vi "Main.vi"() -> ()   [LabVIEW 2019]
uses:
  Type Definitions/Machine States/Signal Playback State.ctl
  Type Definitions/Machine States/Oscillator State.ctl
  Type Definitions/UI.ctl
  Type Definitions/UIOscillatorParam.ctl
  Type Definitions/Sub Oscillalator Type.ctl
  Type Definitions/UIADSRParam.ctl
  Type Definitions/UILowpassParam.ctl
  Type Definitions/UITremolo.ctl
  Type Definitions/DataInOut.ctl
  <vilib>/sound2/lvsound2.llb/Sampling Mode.ctl
  <vilib>/sound2/lvsound2.llb/Sound Data Format.ctl
  <vilib>/sound2/lvsound2.llb/Sound Output Set Volume (Single).vi
  <vilib>/sound2/lvsound2.llb/Sound Output Write (DBL Single).vi
panel:
  in  "Cluster":T1={"oscillator"={"signal type"=0, "pulse width"=0.0, "Sub oscillator"=enum."Off", "Frequency"=0.0, "Amplitude"=0.0}, "ADSR"={"A"=0, "D"=0, "S"=0, "R"=0, "volume"=0.0}, "Lowpass filter"={"Lowpass on/off"=FALSE, "Cutoff frequency"=20.0}, "Tremolo"={"Rate"=0.0, "LFO frequency"=20.0, " on/off "=FALSE}} {"Tremolo"."LFO frequency" min=0.0 max=25.0 scale=0.0..25.0; "Tremolo"."Rate" min=0.0 max=1.0 scale=0.0..1.0; "Lowpass filter"."Cutoff frequency" min=20.0 max=20000.0 scale=20.0..20000.0; "ADSR"."volume" min=0.0 max=100.0 scale=0.0..100.0; "ADSR"."R" scale=0.0..100.0; "ADSR"."S" scale=0.0..100.0; "ADSR"."D" scale=0.0..100.0; "ADSR"."A" scale=0.0..100.0; "oscillator"."Amplitude" scale=0.0..10.0; "oscillator"."Frequency" scale=0.0..10.0; "oscillator"."pulse width" min=0.0 max=100.0 scale=0.0..100.0; "oscillator"."signal type" items=["Sine Wave", "Triangle Wave", "Square Wave", "Sawtooth Wave"]}
  out "Enum":T7
  in  "Sound button":bool
  out "element":waveform(dbl)(graph)
  out "Play State":T8
  out "# elements in queue":i32
  in  "Play Button":bool
  in  "Stop Button":bool
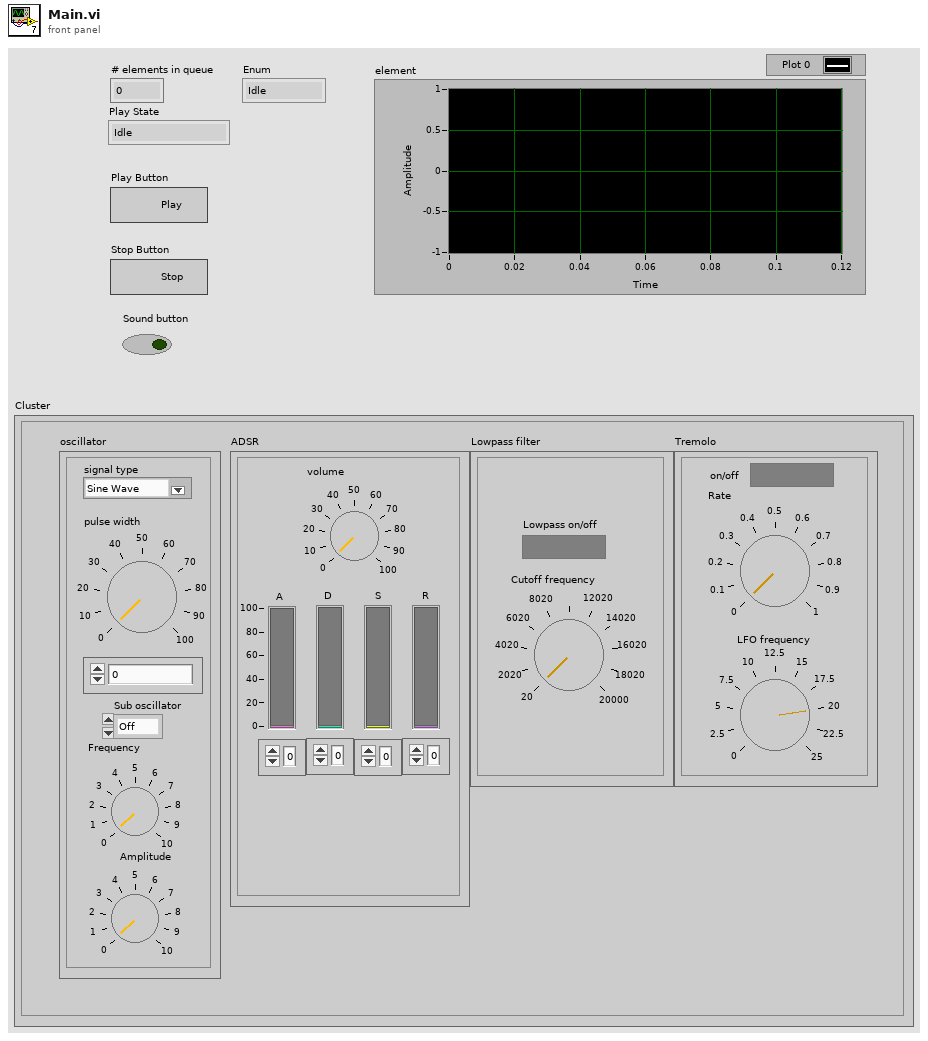
[diagram p1: front panel]
types:
  T1 = typedef "UI.ctl" = cluster{"oscillator":T2, "ADSR":T4, "Lowpass filter":T5, "Tremolo":T6}
  T2 = typedef "UIOscillatorParam.ctl" = cluster{"signal type":u16, "pulse width":dbl, "Sub oscillator":T3, "Frequency":dbl, "Amplitude":dbl}
  T3 = typedef "Sub Oscillalator Type.ctl" = enum16{"Off", "One Octave", "Two Octaves"}
  T4 = typedef "UIADSRParam.ctl" = cluster{"A":i32, "D":i32, "S":i32, "R":i32, "volume":dbl}
  T5 = typedef "UILowpassParam.ctl" = cluster{"Lowpass on/off":bool, "Cutoff frequency":dbl}
  T6 = typedef "UITremolo.ctl" = cluster{"Rate":dbl, "LFO frequency":dbl, " on/off ":bool}
  T7 = typedef "Oscillator State.ctl" = enum16{"Idle", "Attack", "Decay", "Sustain", "Release"}
  T8 = typedef "Signal Playback State.ctl" = enum16{"Idle", "Initialization", "Playing", "End"}
  T9 = typedef "DataInOut.ctl" = enum16{"write", "read"}
  T10 = typedef "Sound Data Format.ctl" = cluster{"sample rate (S/s)":dbl, "number of channels":i32, "bits per sample":i32}
  T11 = typedef "Sampling Mode.ctl" = i32
  T12 = typedef "Sound Output Task ID.ctl" = u32
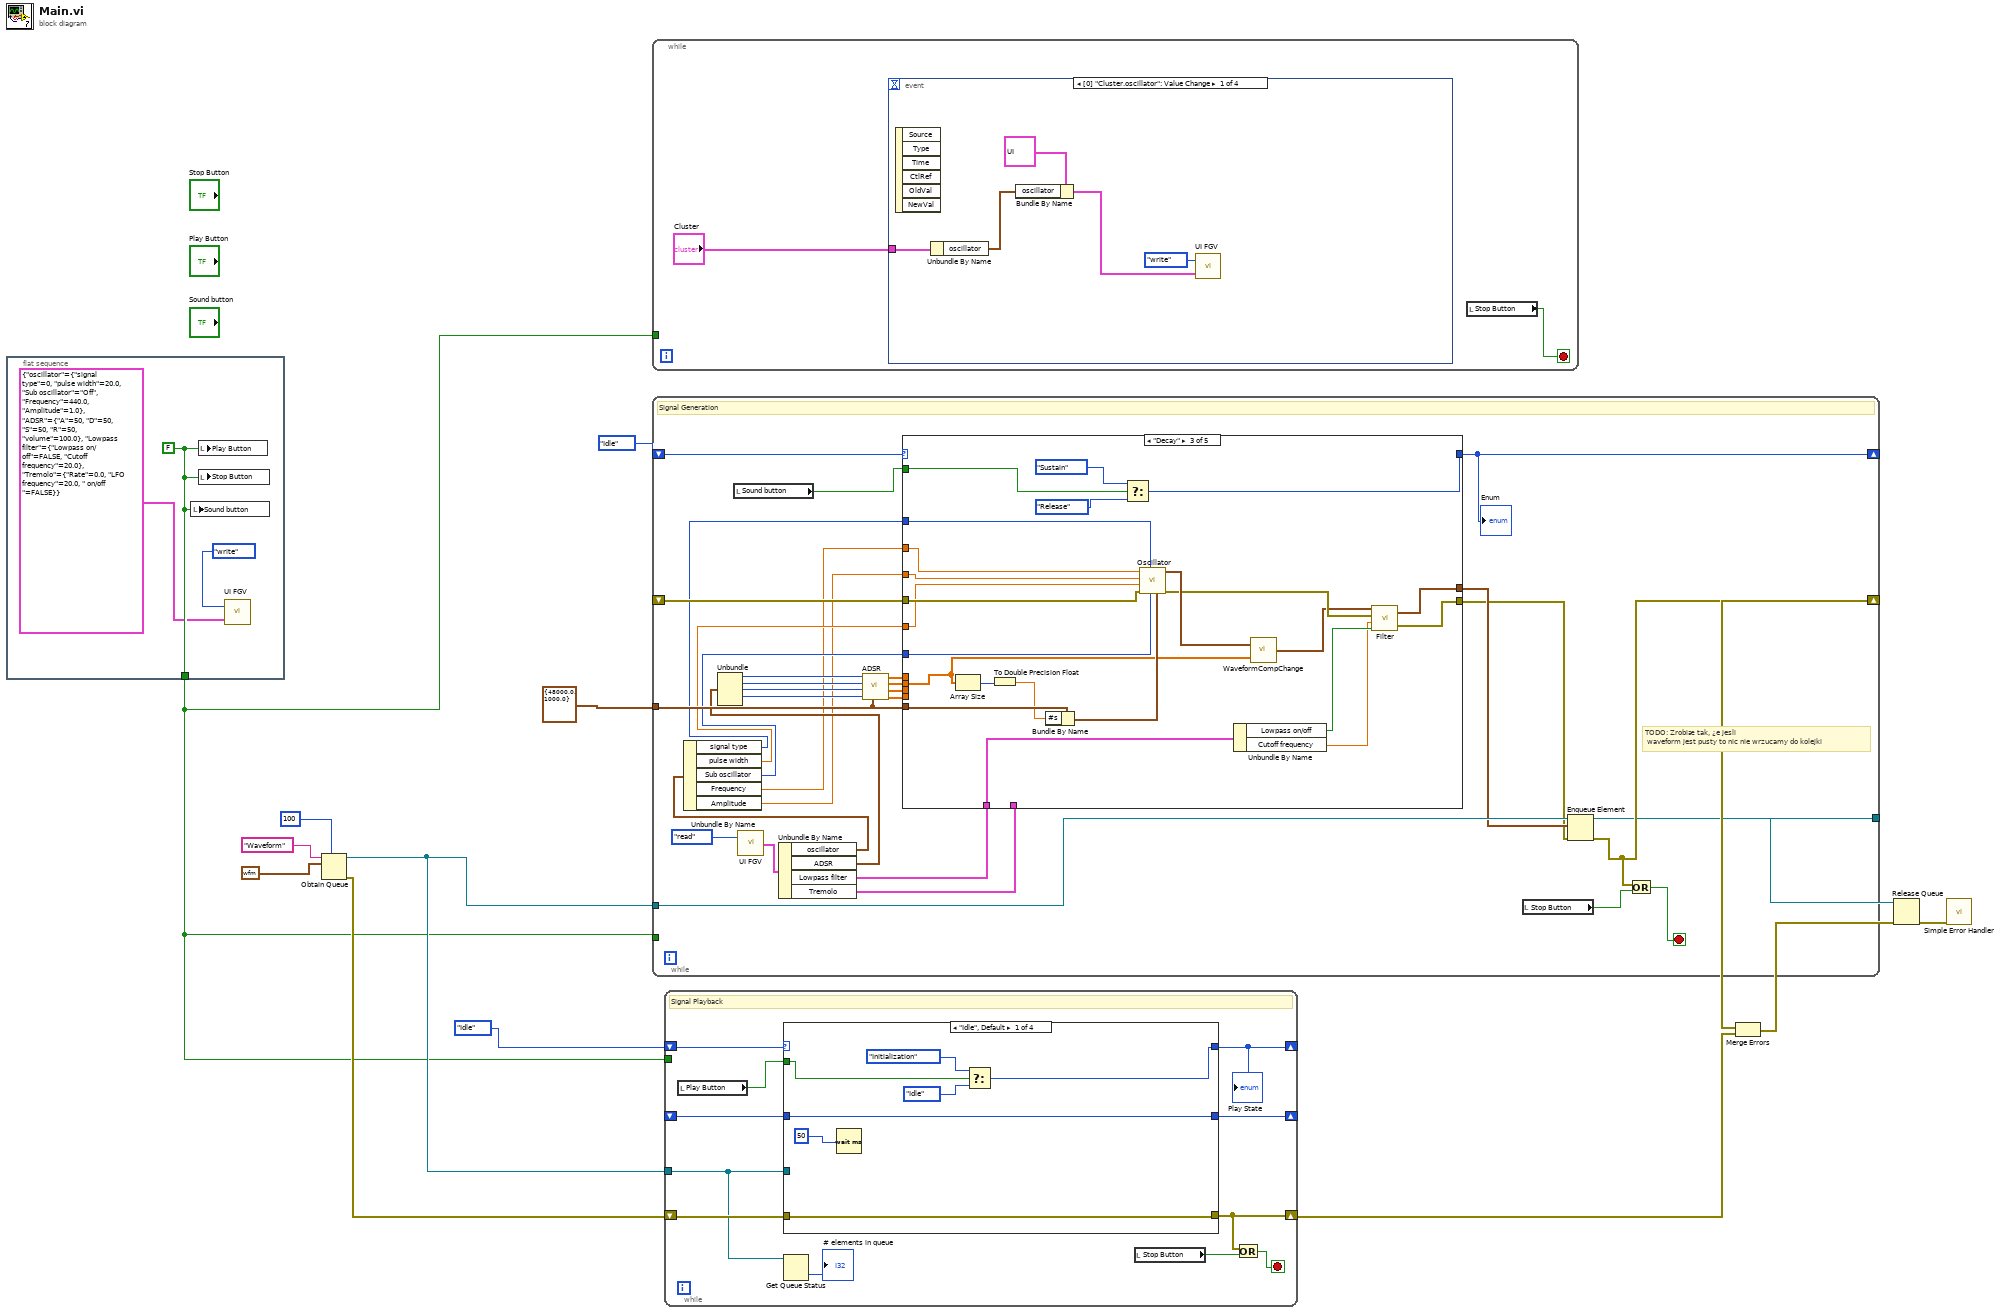
[diagram p0: block diagram]
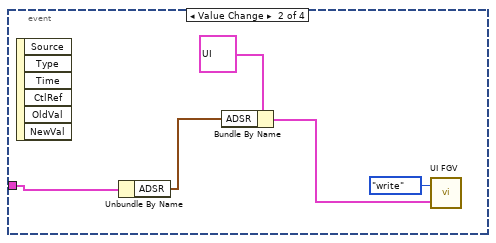
[diagram p2: hidden frame]
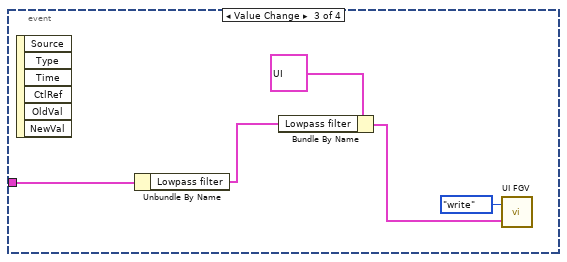
[diagram p3: hidden frame]
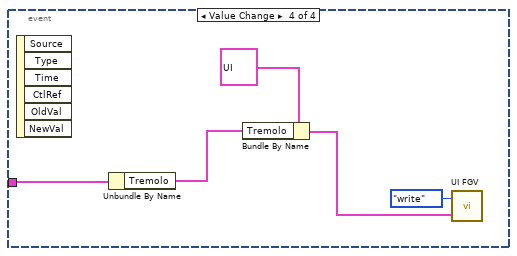
[diagram p4: hidden frame]
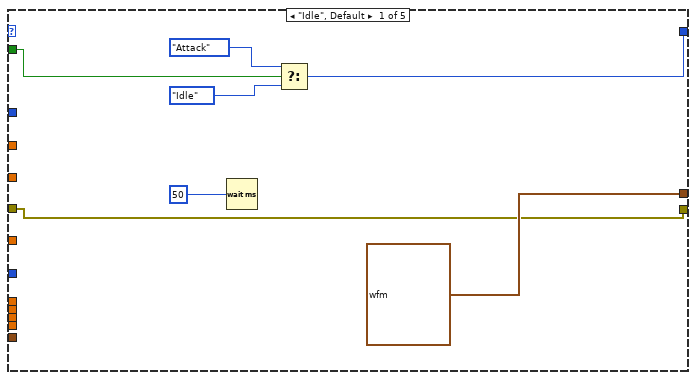
[diagram p5: hidden frame]
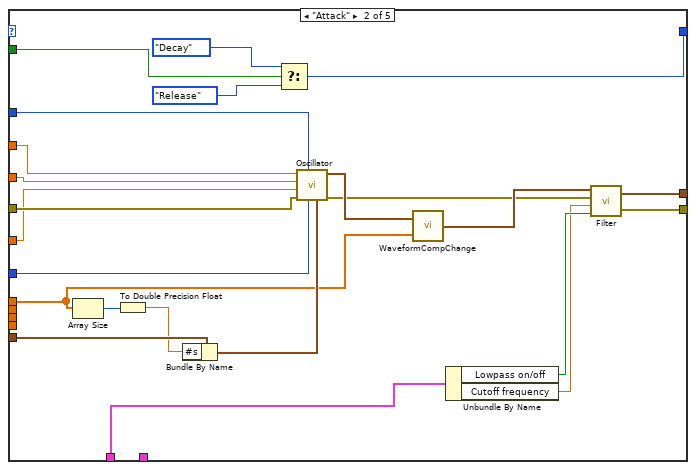
[diagram p6: hidden frame]
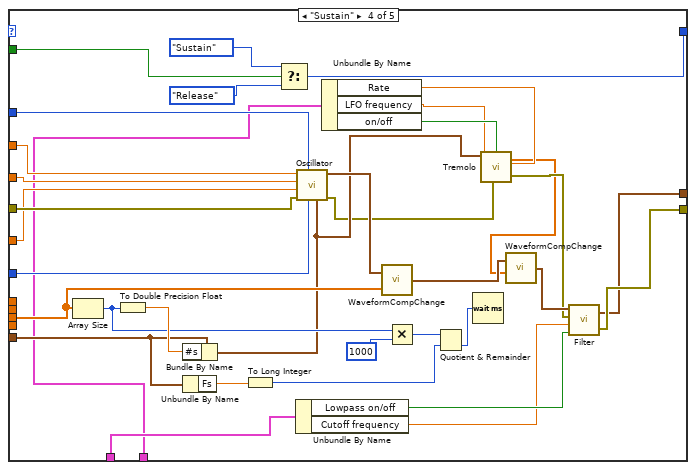
[diagram p7: hidden frame]
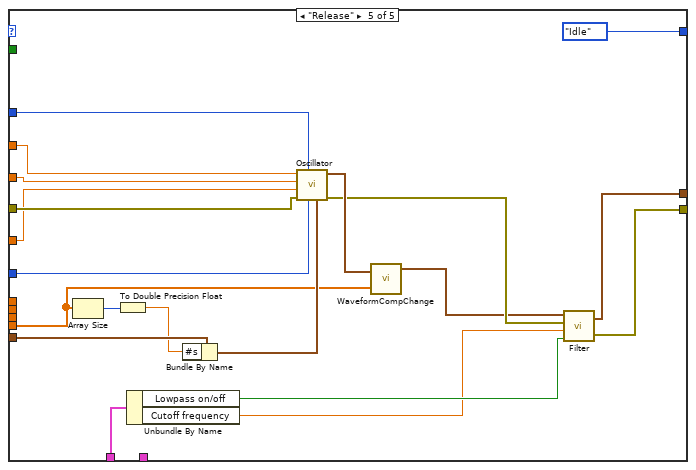
[diagram p8: hidden frame]
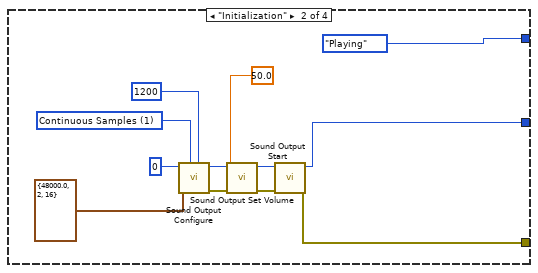
[diagram p9: hidden frame]
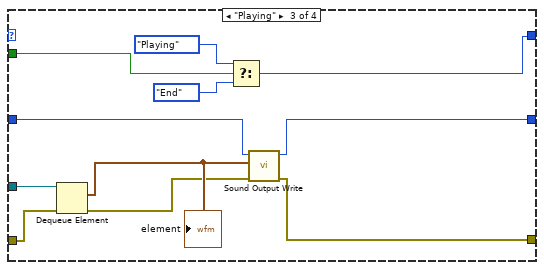
[diagram p10: hidden frame]
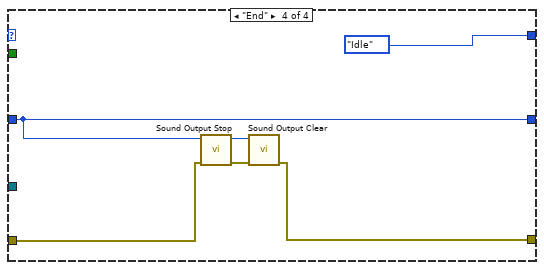
[diagram p11: hidden frame]
diagram:
  n1 = flat-sequence {
    tunnel: [w17] -> w1
    frame #0 {
      w17 = FALSE ("Play Button")
      n2 = local write "Sound button"(w17) -> ()
      n3 = local write "Play Button"(w17) -> ()
      n4 = local write "Stop Button"(w17) -> ()
      n5 = call "UI FGV.vi"("Data in"=T1 {"oscillator"={"signal type"=0, "pulse width"=20.0, "Sub oscillator"=enum."Off", "Frequency"=440.0, "Amplitude"=1.0}, "ADSR"={"A"=50, "D"=50, "S"=50, "R"=50, "volume"=100.0}, "Lowpass filter"={"Lowpass on/off"=FALSE, "Cutoff frequency"=20.0}, "Tremolo"={"Rate"=0.0, "LFO frequency"=20.0, " on/off "=FALSE}}, "Enum"=DataInOut."write") -> ()  [unwired: 1 out]
    }
  }
  n6 = Obtain Queue(max queue size (-1, unlimited)=100, name (unnamed)="Waveform", element data type=waveform(dbl) {"t0"=timestamp(0 s since 1904-01-01), "dt"=1.0, "Y"=[]} ("Waveform out")) -> (queue out=w4:refnum<queue>, error out=w12:errorcluster)  [unwired: 2 in, 1 out]
  n7 = while "User Interface" {
    tunnel: w1 -> [_]
    stop <- w18 stop-if-true
    n8 = event shown="[0] \"Cluster.oscillator\": Value Change" {
      selector: _ -> [_ _ _ _]
      dyn-events: _ -> [_ _ _ _]
      timeout: _ -> [_ _ _ _]
      tunnel: "Cluster" -> [w21 w26 w31 w35]
      event Value Change {
        n9 = event-data() -> ()  [unwired: 1 in, 6 out]
        n10 = Unbundle By Name(w21) -> ("oscillator"=w20:T2)
        n11 = Bundle By Name(cluster=T1 {"oscillator"={"signal type"=0, "pulse width"=0.0, "Sub oscillator"=enum."Off", "Frequency"=0.0, "Amplitude"=0.0}, "ADSR"={"A"=0, "D"=0, "S"=0, "R"=0, "volume"=0.0}, "Lowpass filter"={"Lowpass on/off"=FALSE, "Cutoff frequency"=20.0}, "Tremolo"={"Rate"=0.0, "LFO frequency"=20.0, " on/off "=FALSE}} ("Data in"), "oscillator"=w20) -> (w22:T1)
        n12 = call "UI FGV.vi"("Data in"=w22, "Enum"=DataInOut."write") -> ()  [unwired: 1 out]
      }
      event Value Change {
        n13 = event-data() -> ()  [unwired: 1 in, 6 out]
        n14 = Unbundle By Name(w26) -> ("ADSR"=w25:T4)
        n15 = Bundle By Name(cluster=T1 {"oscillator"={"signal type"=0, "pulse width"=0.0, "Sub oscillator"=enum."Off", "Frequency"=0.0, "Amplitude"=0.0}, "ADSR"={"A"=0, "D"=0, "S"=0, "R"=0, "volume"=0.0}, "Lowpass filter"={"Lowpass on/off"=FALSE, "Cutoff frequency"=20.0}, "Tremolo"={"Rate"=0.0, "LFO frequency"=20.0, " on/off "=FALSE}} ("Data in"), "ADSR"=w25) -> (w27:T1)
        n16 = call "UI FGV.vi"("Data in"=w27, "Enum"=DataInOut."write") -> ()  [unwired: 1 out]
      }
      event Value Change {
        n17 = event-data() -> ()  [unwired: 1 in, 6 out]
        n18 = Unbundle By Name(w31) -> ("Lowpass filter"=w30:T5)
        n19 = Bundle By Name(cluster=T1 {"oscillator"={"signal type"=0, "pulse width"=0.0, "Sub oscillator"=enum."Off", "Frequency"=0.0, "Amplitude"=0.0}, "ADSR"={"A"=0, "D"=0, "S"=0, "R"=0, "volume"=0.0}, "Lowpass filter"={"Lowpass on/off"=FALSE, "Cutoff frequency"=20.0}, "Tremolo"={"Rate"=0.0, "LFO frequency"=20.0, " on/off "=FALSE}} ("Data in"), "Lowpass filter"=w30) -> (w32:T1)
        n20 = call "UI FGV.vi"("Data in"=w32, "Enum"=DataInOut."write") -> ()  [unwired: 1 out]
      }
      event Value Change {
        n21 = event-data() -> ()  [unwired: 1 in, 6 out]
        n22 = Unbundle By Name(w35) -> ("Tremolo"=w36:T6)
        n23 = Bundle By Name(cluster=T1 {"oscillator"={"signal type"=0, "pulse width"=0.0, "Sub oscillator"=enum."Off", "Frequency"=0.0, "Amplitude"=0.0}, "ADSR"={"A"=0, "D"=0, "S"=0, "R"=0, "volume"=0.0}, "Lowpass filter"={"Lowpass on/off"=FALSE, "Cutoff frequency"=20.0}, "Tremolo"={"Rate"=0.0, "LFO frequency"=20.0, " on/off "=FALSE}} ("Data in"), "Tremolo"=w36) -> (w37:T1)
        n24 = call "UI FGV.vi"("Data in"=w37, "Enum"=DataInOut."write") -> ()  [unwired: 1 out]
      }
    }
    n25 = local read "Stop Button"() -> (w18:bool)
  }
  n26 = while {
    shift-right: [w68] -> _
    shift-left: Oscillator_State."Idle" -> [w70]
    tunnel: cluster{"Fs":dbl, "#s":dbl} {"Fs"=48000.0, "#s"=1000.0} ("Sampling info") -> [w62]
    shift-right: [w64] -> w2
    shift-left: _ -> [w69]
    tunnel: w1 -> [_]
    tunnel: w4 -> [w53]
    tunnel: [w63] -> w3
    stop <- w65 stop-if-true
    # "TODO: Zrobiæ tak, ¿e jesli\n waveform jest pusty to nic nie wrzucamy do kolejki"
    # "Signal Generation"
    n27 = local read "Sound button"() -> (w67:bool)
    n28 = call "UI FGV.vi"("Enum"=DataInOut."read") -> ("Data out"=w49:T1)  [unwired: 1 in]
    n29 = Unbundle By Name(w49) -> ("oscillator"=w48:T2, "ADSR"=w44:T4, "Lowpass filter"=w43:T5, "Tremolo"=w42:T6)
    n30 = Unbundle By Name(w48) -> ("signal type"=w47:u16, "pulse width"=w46:dbl, "Sub oscillator"=w45:T3, "Frequency"=w41:dbl, "Amplitude"=w40:dbl)
    n31 = Unbundle(w44) -> ("A"=w61:i32, "D"=w60:i32, "S"=w59:i32, "R"=w58:i32)  [unwired: 1 out]
    n32 = call "ADSR.vi"("Sampling info"=w62, "R"=w58, "S"=w59, "D"=w60, "A"=w61) -> ("R"=w54:dbl[], "S"=w55:dbl[], "D"=w56:dbl[], "A"=w57:dbl[])  [unwired: 3 in]
    n33 = case shown="\"Decay\"" w70 {
      tunnel: [w75 w99 w121 w156 Oscillator_State."Idle"] -> w68
      tunnel: w67 -> [w73 w98 w120 w155 _]
      tunnel: w47 -> [_ w92 w114 w149 w173]
      tunnel: w41 -> [_ w93 w115 w150 w174]
      tunnel: w40 -> [_ w94 w116 w151 w175]
      tunnel: w69 -> [w71 w97 w119 w154 w178]
      tunnel: w46 -> [_ w96 w118 w153 w177]
      tunnel: w45 -> [_ w95 w117 w152 w176]
      tunnel: w62 -> [_ w91 w113 w145 w172]
      tunnel: [w71 w79 w102 w132 w159] -> w51
      tunnel: [waveform(dbl) {"t0"=timestamp(0 s since 1904-01-01), "dt"=1.0, "Y"=[]} ("signal out") w78 w101 w131 w160] -> w52
      tunnel: w57 -> [_ w86 _ _ _]
      tunnel: w56 -> [_ _ w108 _ _]
      tunnel: w55 -> [_ _ _ w139 _]
      tunnel: w54 -> [_ _ _ _ w166]
      tunnel: w43 -> [_ w84 w107 w137 w165]
      tunnel: w42 -> [_ _ _ w136 _]
      frame "Idle", Default {
        n34 = Wait (ms)(milliseconds to wait=u32 50) -> ()  [unwired: 1 out]
        n35 = Select(t=Oscillator_State."Attack", s=w73, f=Oscillator_State."Idle") -> (s? t:f=w75:T7)
      }
      frame "Attack" {
        n36 = Array Size(array=w86) -> (size(s)=w90:i32)
        n37 = To Double Precision Float(number=w90) -> (double precision float=w89:dbl)
        n38 = Bundle By Name(cluster=w91, "#s"=w89) -> (w88:cluster{"Fs":dbl, "#s":dbl})
        n39 = Select(t=Oscillator_State."Decay", s=w98, f=Oscillator_State."Release") -> (s? t:f=w99:T7)
        n40 = call "Oscillator.vi"("Sampling info"=w88, "Sub Oscillator Type"=w95, "Waveform type"=w92, "Error in"=w97, "Pulse Width"=w96, "Amplitude"=w94, "Frequency"=w93) -> ("Error out"=w80:errorcluster, "Waveform out"=w85:waveform(dbl))  [unwired: 3 in]
        n41 = call "WaveformCompChange.vi"("component"=w86, "input waveform"=w85) -> ("output waveform"=w81:waveform(dbl))
        n42 = Unbundle By Name(w84) -> ("Lowpass on/off"=w83:bool, "Cutoff frequency"=w82:dbl)
        n43 = call "Filter.vi"("on/off"=w83, "Cutoff freq (Hz)"=w82, "error in"=w80, "signal in"=w81) -> ("error out"=w79:errorcluster, "signal out"=w78:waveform(dbl))
      }
      frame "Decay" {
        n44 = Array Size(array=w108) -> (size(s)=w112:i32)
        n45 = To Double Precision Float(number=w112) -> (double precision float=w111:dbl)
        n46 = Bundle By Name(cluster=w113, "#s"=w111) -> (w110:cluster{"Fs":dbl, "#s":dbl})
        n47 = Select(t=Oscillator_State."Sustain", s=w120, f=Oscillator_State."Release") -> (s? t:f=w121:T7)
        n48 = call "Oscillator.vi"("Sampling info"=w110, "Sub Oscillator Type"=w117, "Waveform type"=w114, "Error in"=w119, "Pulse Width"=w118, "Amplitude"=w116, "Frequency"=w115) -> ("Error out"=w104:errorcluster, "Waveform out"=w109:waveform(dbl))  [unwired: 3 in]
        n49 = Unbundle By Name(w107) -> ("Lowpass on/off"=w106:bool, "Cutoff frequency"=w105:dbl)
        n50 = call "WaveformCompChange.vi"("component"=w108, "input waveform"=w109) -> ("output waveform"=w103:waveform(dbl))
        n51 = call "Filter.vi"("on/off"=w106, "Cutoff freq (Hz)"=w105, "error in"=w104, "signal in"=w103) -> ("error out"=w102:errorcluster, "signal out"=w101:waveform(dbl))
      }
      frame "Sustain" {
        n52 = Array Size(array=w139) -> (size(s)=w147:i32)
        n53 = To Double Precision Float(number=w147) -> (double precision float=w148:dbl)
        n54 = Bundle By Name(cluster=w145, "#s"=w148) -> (w127:cluster{"Fs":dbl, "#s":dbl})
        n55 = Unbundle By Name(w145) -> ("Fs"=w144:dbl)
        n56 = To Long Integer(number=w144) -> (32bit integer=w142:i32)
        n57 = Select(t=Oscillator_State."Sustain", s=w155, f=Oscillator_State."Release") -> (s? t:f=w156:T7)
        n58 = Unbundle By Name(w137) -> ("Lowpass on/off"=w134:bool, "Cutoff frequency"=w133:dbl)
        n59 = call "Oscillator.vi"("Sampling info"=w127, "Sub Oscillator Type"=w152, "Waveform type"=w149, "Error in"=w154, "Pulse Width"=w153, "Amplitude"=w151, "Frequency"=w150) -> ("Error out"=w126:errorcluster, "Waveform out"=w140:waveform(dbl))  [unwired: 3 in]
        n60 = Unbundle By Name(w136) -> ("Rate"=w128:dbl, "LFO frequency"=w129:dbl, "on/off"=w130:bool)
        n61 = call "WaveformCompChange.vi"("component"=w139, "input waveform"=w140) -> ("output waveform"=w138:waveform(dbl))
        n62 = Multiply(x=w147, y=1000) -> (x*y=w143:i32)
        n63 = Quotient & Remainder(x=w143, y=w142) -> (floor(x/y)=w141:i32)  [unwired: 1 out]
        n64 = Wait (ms)(milliseconds to wait=w141) -> ()  [unwired: 1 out]
        n65 = call "Tremolo.vi"("sampling info"=w127, "amplitude"=w128, "frequency"=w129, "on/off"=w130, "error in"=w126) -> ("signal out"=w124:dbl[], "error out"=w125:errorcluster)
        n66 = call "WaveformCompChange.vi"("component"=w124, "input waveform"=w138) -> ("output waveform"=w135:waveform(dbl))
        n67 = call "Filter.vi"("on/off"=w134, "Cutoff freq (Hz)"=w133, "error in"=w125, "signal in"=w135) -> ("error out"=w132:errorcluster, "signal out"=w131:waveform(dbl))
      }
      frame "Release" {
        n68 = Array Size(array=w166) -> (size(s)=w171:i32)
        n69 = To Double Precision Float(number=w171) -> (double precision float=w170:dbl)
        n70 = Unbundle By Name(w165) -> ("Lowpass on/off"=w164:bool, "Cutoff frequency"=w163:dbl)
        n71 = Bundle By Name(cluster=w172, "#s"=w170) -> (w169:cluster{"Fs":dbl, "#s":dbl})
        n72 = call "Oscillator.vi"("Sampling info"=w169, "Sub Oscillator Type"=w176, "Waveform type"=w173, "Error in"=w178, "Pulse Width"=w177, "Amplitude"=w175, "Frequency"=w174) -> ("Error out"=w162:errorcluster, "Waveform out"=w167:waveform(dbl))  [unwired: 3 in]
        n73 = call "WaveformCompChange.vi"("component"=w166, "input waveform"=w167) -> ("output waveform"=w161:waveform(dbl))
        n74 = call "Filter.vi"("on/off"=w164, "Cutoff freq (Hz)"=w163, "error in"=w162, "signal in"=w161) -> ("error out"=w159:errorcluster, "signal out"=w160:waveform(dbl))
      }
    }
    "Enum" <- w68
    n75 = local read "Stop Button"() -> (w66:bool)
    n76 = Enqueue Element(queue=w53, element=w52, error in (no error)=w51) -> (queue out=w63:refnum<queue>, error out=w64:errorcluster)  [unwired: 1 in, 1 out]
    n77 = Or(x=w64, y=w66) -> (x .or. y?=w65:bool)
  }
  n78 = while {
    shift-right: [w184] -> w10
    shift-left: w12 -> [w188]
    shift-right: [w187] -> _
    shift-left: Signal_Playback_State."Idle" -> [w189]
    shift-right: [w183] -> _
    shift-left: _ -> [w186]
    tunnel: w4 -> [w180]
    tunnel: w1 -> [_]
    stop <- w185 stop-if-true
    # "Signal Playback"
    n79 = local read "Play Button"() -> (w182:bool)
    n80 = case shown="\"Idle\", Default" w189 {
      tunnel: [w196 w200 w211 w221] -> w184
      tunnel: w188 -> [w196 _ w219 w222]
      tunnel: w182 -> [w190 _ w209 _]
      tunnel: [w193 Signal_Playback_State."Playing" ("f") w218 Signal_Playback_State."Idle" ("f")] -> w187
      tunnel: w186 -> [w191 _ w214 w220]
      tunnel: w180 -> [_ _ w210 _]
      tunnel: [w191 w199 w213 w220] -> w183
      frame "Idle", Default {
        n81 = Wait (ms)(milliseconds to wait=u32 50) -> ()  [unwired: 1 out]
        n82 = Select(t=Signal_Playback_State."Initialization", s=w190, f=Signal_Playback_State."Idle") -> (s? t:f=w193:T8)
      }
      frame "Initialization" {
        w202 = T11 1 items=["Finite Samples", "Continuous Samples"] ("sample mode")
        n83 = call <vilib>:"Sound Output Configure.vi"("number of samples/ch"=1200, "sample mode"=w202, "sound format"=T10 {"sample rate (S/s)"=48000.0, "number of channels"=2, "bits per sample"=16}, "device ID"=u32 0) -> ("error out"=w204:errorcluster, "task ID"=w205:T12)  [unwired: 6 in]
        n84 = call-poly <vilib>:"Sound Output Set Volume.vi"("error in (no error)"=w204, "volume"=50.0, "task ID"=w205) -> ("error out"=w207:errorcluster, "task ID out"=w206:T12)  [unwired: 7 in]
        n85 = call <vilib>:"Sound Output Start.vi"("error in (no error)"=w207, "task ID"=w206) -> ("error out"=w200:errorcluster, "task ID out"=w199:T12)  [unwired: 8 in]
      }
      frame "Playing" {
        n86 = Dequeue Element(queue=w210, error in (no error)=w219) -> (element=w215:waveform(dbl), error out=w212:errorcluster)  [unwired: 1 in, 2 out]
        "element" <- w215
        n87 = Select(t=Signal_Playback_State."Playing", s=w209, f=Signal_Playback_State."End") -> (s? t:f=w218:T8)
        n88 = call-poly <vilib>:"Sound Output Write.vi"("error in (no error)"=w212, "data"=w215, "task ID"=w214) -> ("error out"=w211:errorcluster, "task ID out"=w213:T12)  [unwired: 7 in]
      }
      frame "End" {
        n89 = call <vilib>:"Sound Output Stop.vi"("error in (no error)"=w222, "task ID"=w220) -> ("error out"=w223:errorcluster, "task ID out"=w224:T12)  [unwired: 8 in]
        n90 = call <vilib>:"Sound Output Clear.vi"("error in (no error)"=w223, "task ID"=w224) -> ("error out"=w221:errorcluster)  [unwired: 9 in]
      }
    }
    "Play State" <- w187
    n91 = Get Queue Status(queue=w180) -> (# elements in queue=→"# elements in queue":i32)  [unwired: 2 in, 7 out]
    n92 = local read "Stop Button"() -> (w181:bool)
    n93 = Or(x=w184, y=w181) -> (x .or. y?=w185:bool)
  }
  n94 = Merge Errors(w2, w10) -> (w7:errorcluster)
  n95 = Release Queue(queue=w3, error in (no error)=w7) -> (error out=w8:errorcluster)  [unwired: 1 in, 2 out]
  n96 = call <vilib>:"Simple Error Handler.vi"("error in (no error)"=w8) -> ()  [unwired: 4 in, 5 out]
